vi "Reset Abort.vi"(8 "error in (no error)":errorcluster, 11 "AbortManager in":refnum<class "AbortManager.lvclass">) -> (0 "error out":errorcluster, 3 "AbortManager out":refnum<class "AbortManager.lvclass">)   [LabVIEW 2020, in "Volatus.lvlib" / "AbortManager.lvclass"]
uses:
  AbortManager.lvclass
  AbortManager.lvclass/AbortManager.ctl
  AbortHandler Messages/Reset Abort Msg/Reset Abort Msg.lvclass
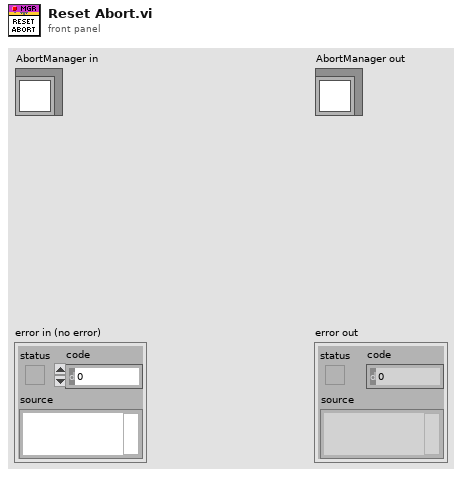
[diagram p1: front panel]
types:
  T1 = map{string, refnum<class "Message Enqueuer.lvclass">}
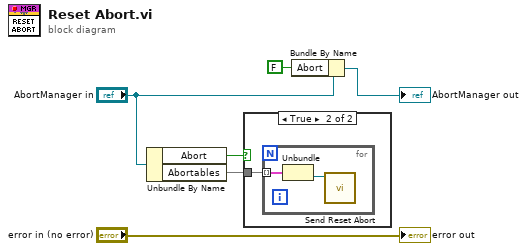
[diagram p0: block diagram]
diagram:
  n1 = Unbundle By Name("AbortManager in") -> ("Abort"=w1:bool, "Abortables"=w5:T1)
  n2 = case shown="True" w1 {
    tunnel: w5 -> [_ w7]
    frame False {
    }
    frame True {
      n3 = for {
        tunnel: w7 -> [w9] mode=indexing
        n4 = Unbundle(w9) -> ("EnQr"=w8:refnum<class "Message Enqueuer.lvclass">)  [unwired: 1 out]
        n5 = call "Send Reset Abort.vi"("Message Enqueuer"=w8) -> ()  [unwired: 9 in, 2 out]
      }
    }
  }
  n6 = Bundle By Name(cluster="AbortManager in", "Abort"=FALSE) -> (→"AbortManager out":refnum<class "AbortManager.lvclass">)
  "error out" <- "error in (no error)"
